vi "VI Tree.vi"   [LabVIEW 2015, in "LeCroy Wave Series.lvlib"]
doc: "This is the instrument driver for the LeCroy Wave Series Oscilloscopes. The VI Tree displays all the user-callable VIs of the instrument driver in an organized table."
uses:
  <instrlib>/LeCroy Wave Series/LeCroy Wave Series.lvlib
  <instrlib>/LeCroy Wave Series/Public/Data/Read Single Waveform.vi
  <instrlib>/LeCroy Wave Series/Public/Configure/Configure Edge Trigger.vi
  <instrlib>/LeCroy Wave Series/Public/Data/Read Waveform Measurement (Standard).vi
panel:
  # "(c) 2008 - 2012 NATIONAL INSTRUMENTS.  ALL RIGHTS RESERVED."
  # "SEE DIAGRAM\nFOR VI TREE."
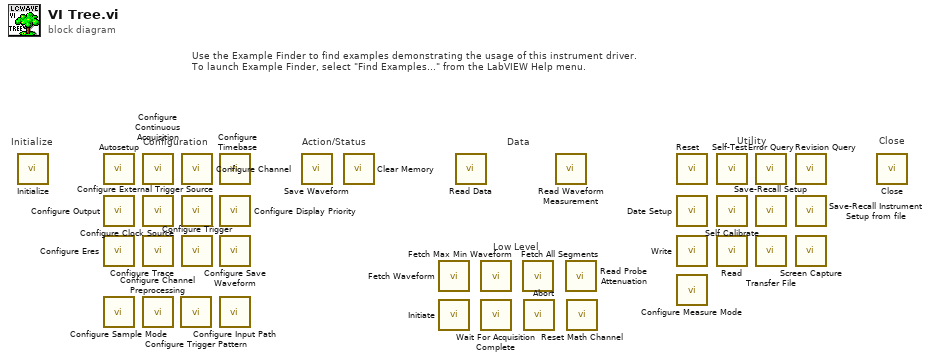
[diagram p0: block diagram]
diagram:
  # "Low Level"
  # "Action/Status"
  # "Use the Example Finder to find examples demonstrating the usage of this instrument driver.\nTo launch Example Finder, select \"Find Examples...\" from the LabVIEW Help menu."
  # "Configuration"
  # "Utility"
  # "Data"
  # "Close"
  # "Initialize"
  n1 = call <instrlib>:"Initialize.vi"() -> ()  [unwired: 10 in, 2 out]
  n2 = call <instrlib>:"Autosetup.vi"() -> ()  [unwired: 10 in, 2 out]
  n3 = call <instrlib>:"Configure Output.vi"() -> ()  [unwired: 14 in, 2 out]
  n4 = call <instrlib>:"Configure Eres.vi"() -> ()  [unwired: 10 in, 2 out]
  n5 = call <instrlib>:"Configure Sample Mode.vi"() -> ()  [unwired: 10 in, 2 out]
  n6 = call <instrlib>:"Configure Continuous Acquisition.vi"() -> ()  [unwired: 10 in, 2 out]
  n7 = call <instrlib>:"Configure Clock Source.vi"() -> ()  [unwired: 10 in, 2 out]
  n8 = call <instrlib>:"Configure Trace.vi"() -> ()  [unwired: 10 in, 2 out]
  n9 = call <instrlib>:"Configure Channel Preprocessing.vi"() -> ()  [unwired: 14 in, 2 out]
  n10 = call <instrlib>:"Configure Trigger Pattern.vi"() -> ()  [unwired: 18 in, 2 out]
  n11 = call <instrlib>:"Configure Channel.vi"() -> ()  [unwired: 14 in, 2 out]
  n12 = call <instrlib>:"Configure External Trigger Source.vi"() -> ()  [unwired: 10 in, 2 out]
  n13 = call-poly <instrlib>:"Configure Trigger.vi"() -> ()  [unwired: 14 in, 2 out]
  n14 = call <instrlib>:"Configure Timebase.vi"() -> ()  [unwired: 10 in, 2 out]
  n15 = call <instrlib>:"Configure Display Priority.vi"() -> ()  [unwired: 10 in, 2 out]
  n16 = call <instrlib>:"Configure Save Waveform.vi"() -> ()  [unwired: 18 in, 2 out]
  n17 = call <instrlib>:"Configure Input Path.vi"() -> ()  [unwired: 14 in, 2 out]
  n18 = call <instrlib>:"Save Waveform.vi"() -> ()  [unwired: 9 in, 3 out]
  n19 = call <instrlib>:"Clear Memory.vi"() -> ()  [unwired: 10 in, 2 out]
  n20 = call <instrlib>:"Fetch Waveform.vi"() -> ()  [unwired: 9 in, 3 out]
  n21 = call <instrlib>:"Initiate.vi"() -> ()  [unwired: 10 in, 2 out]
  n22 = call-poly <instrlib>:"Read Data.vi"() -> ()  [unwired: 9 in, 3 out]
  n23 = call <instrlib>:"Fetch Max Min Waveform.vi"() -> ()  [unwired: 8 in, 4 out]
  n24 = call <instrlib>:"Wait For Acquisition Complete.vi"() -> ()  [unwired: 9 in, 3 out]
  n25 = call <instrlib>:"Fetch All Segments.vi"() -> ()  [unwired: 9 in, 3 out]
  n26 = call <instrlib>:"Abort.vi"() -> ()  [unwired: 10 in, 2 out]
  n27 = call-poly <instrlib>:"Read Waveform Measurement.vi"() -> ()  [unwired: 12 in, 4 out]
  n28 = call <instrlib>:"Read Probe Attenuation.vi"() -> ()  [unwired: 9 in, 3 out]
  n29 = call <instrlib>:"Reset Math Channel.vi"() -> ()  [unwired: 10 in, 2 out]
  n30 = call <instrlib>:"Reset.vi"() -> ()  [unwired: 10 in, 2 out]
  n31 = call <instrlib>:"Date Setup.vi"() -> ()  [unwired: 14 in, 2 out]
  n32 = call <instrlib>:"Write.vi"() -> ()  [unwired: 9 in, 3 out]
  n33 = call <instrlib>:"Configure Measure Mode.vi"() -> ()  [unwired: 14 in, 2 out]
  n34 = call <instrlib>:"Self-Test.vi"() -> ()  [unwired: 8 in, 4 out]
  n35 = call <instrlib>:"Self Calibrate.vi"() -> ()  [unwired: 10 in, 2 out]
  n36 = call <instrlib>:"Read.vi"() -> ()  [unwired: 8 in, 4 out]
  n37 = call <instrlib>:"Error Query.vi"() -> ()  [unwired: 8 in, 4 out]
  n38 = call <instrlib>:"Save-Recall Setup.vi"() -> ()  [unwired: 10 in, 2 out]
  n39 = call <instrlib>:"Transfer File.vi"() -> ()  [unwired: 10 in, 2 out]
  n40 = call <instrlib>:"Revision Query.vi"() -> ()  [unwired: 8 in, 4 out]
  n41 = call <instrlib>:"Save-Recall Instrument Setup from file.vi"() -> ()  [unwired: 14 in, 2 out]
  n42 = call <instrlib>:"Screen Capture.vi"() -> ()  [unwired: 10 in, 2 out]
  n43 = call <instrlib>:"Close.vi"() -> ()  [unwired: 11 in, 1 out]
